vi "Write Crosshead Status.vi"(8 "error in (no error)":errorcluster, 10 "Crosshead Status":T1, 11 "Force Test Stand in":refnum<class "Force Test Stand.lvclass">) -> (0 "error out":errorcluster, 3 "Force Test Stand out":refnum<class "Force Test Stand.lvclass">)   [LabVIEW 2018, in "Force Test Stand.lvlib" / "Force Test Stand.lvclass"]
uses:
  Force Test Stand.lvclass
  Custom Controls/Crosshead Status.ctl
  Force Test Stand.lvclass/Force Test Stand.ctl
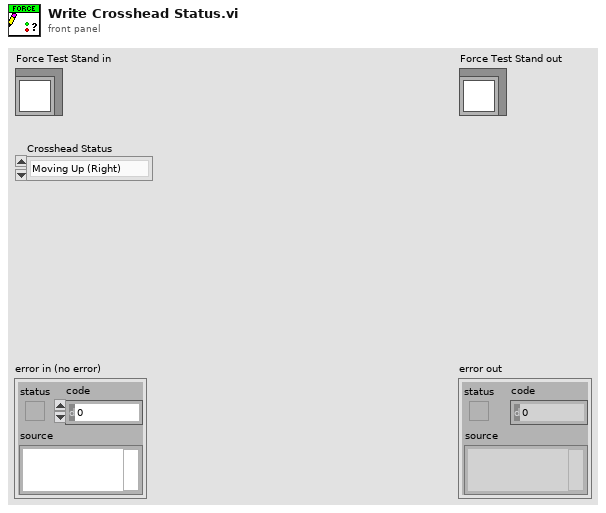
[diagram p1: front panel]
types:
  T1 = typedef "Force Test Stand.lvlib/Force Test Stand.lvclass/Crosshead Status.ctl" = enum16{"Moving Up (Right)", "Moving Down (Left)", "Stopped"}
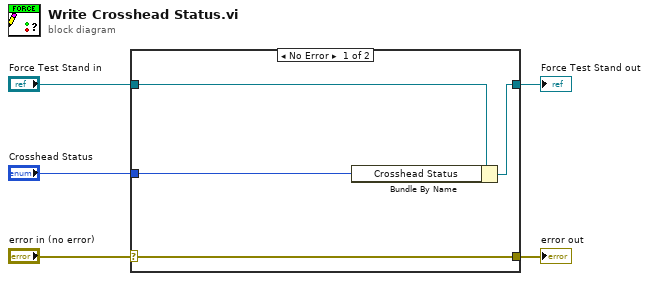
[diagram p0: block diagram]
diagram:
  n1 = case shown="No Error" "error in (no error)" {
    selector: "error in (no error)" -> [w9 w10]
    tunnel: [w9 w10] -> w4
    tunnel: [w7 w11] -> w2
    tunnel: "Force Test Stand in" -> [w8 w11]
    tunnel: "Crosshead Status" -> [w6 _]
    frame No Error {
      n2 = Bundle By Name(cluster=w8, "Crosshead Status"=w6) -> (w7:refnum<class "Force Test Stand.lvclass">)
    }
    frame Error {
    }
  }
  "error out" <- w4
  "Force Test Stand out" <- w2
